vi "MENU1.vi"   [LabVIEW 2020, in "Lazyboots Menu Tool Launch.lvlib"]
uses:
  _Library/Lazyboots Menu Tool Launch.lvlib
  <vilib>/Utility/config.llb/Read Key (String).vi
  <vilib>/Utility/config.llb/NI_LVConfig.lvlib
panel:
  # "Launching..."
types:
  T1 = enum32{"Invalid", "Standard", "Closed", "Hidden", "Minimized", "Maximized"}
  T2 = typedef "NI_LVConfig.lvlib/Config Data RefNum.ctl" = refnum<k1>
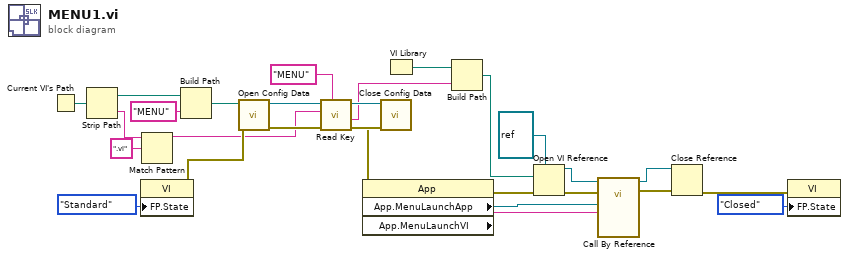
[diagram p0: block diagram]
diagram:
  n1 = Current VI's Path() -> (path=w20:path)
  n2 = Strip Path(path=w20) -> (stripped path=w19:path, name=w9:string)
  n3 = property class="VI"("FP.State"=T1."Standard" ("Front Panel Window:State")) -> (error out=w11:errorcluster)  [unwired: 2 in, 1 out]
  n4 = Match Pattern(string=w9, regular expression=".vi") -> (before substring=w8:string)  [unwired: 4 out]
  n5 = Build Path(base path=w19, name or relative path="MENU") -> (appended path=w17:path)
  n6 = call <vilib>:"Open Config Data.vi"("error in (no error)"=w11, "configuration file path"=w17) -> ("error out"=w15:errorcluster, "refnum"=w16:T2)  [unwired: 7 in, 1 out]
  n7 = call-poly <vilib>:"Read Key.vi"("section"="MENU", "error in (no error)"=w15, "key"=w8, "refnum"=w16) -> ("error out"=w12:errorcluster, "value"=w5:string, "refnum out"=w13:T2)  [unwired: 2 in, 3 out]
  n8 = call <vilib>:"Close Config Data.vi"("error in (no error)"=w12, "refnum"=w13) -> ("error out"=w10:errorcluster)  [unwired: 1 in, 8 out]
  n9 = property class="App"(error in=w10) -> (error out=w25:errorcluster, "App.MenuLaunchApp"=w2:refnum<vi>, "App.MenuLaunchVI"=w1:string)  [unwired: 1 in, 1 out]
  n10 = VI Library() -> (path=w4:path)
  n11 = Build Path(base path=w4, name or relative path=w5) -> (appended path=w6:path)
  n12 = Open VI Reference(type specifier VI Refnum (for type only)=refnum<vi> refnum, vi path=w6, error in (no error)=w25) -> (vi reference=w3:refnum<vi>, error out=w24:errorcluster)  [unwired: 3 out]
  n13 = call-by-ref "?"(reference=w3, error in=w24, "VI Path"=w1, "Application Reference"=w2) -> (reference out=w23:refnum<vi>, error out=w22:errorcluster)  [unwired: 9 in, 1 out]
  n14 = Close Reference(reference=w23, error in (no error)=w22) -> (error out=w21:errorcluster)
  n15 = property class="VI"(error in=w21, "FP.State"=T1."Closed" ("Front Panel Window:State")) -> ()  [unwired: 1 in, 2 out]
